vi "TRIG_CHAN_AUX_HAND.vi"(0 "VISA IN":refnum<visa-resource-name>, 1 "Aux":i32, 2 "Handshake":bool, 5 "error in":errorcluster, 7 "Channel":i32) -> (14 "VISA Out":refnum<visa-resource-name>, 19 "error out":errorcluster)   [LabVIEW 2018, in "PNA-X.lvlib"]
doc: "TRIGger:CHANnel<ch>:AUX<n>:HANDshake <bool> \n(Read-Write) Turns handshake ON / OFF. \nTo enable handshake, the main trigger enable must also be set using TRIG:CHAN:AUX:ENAB. \nWhen ON, PNA waits indefinitely for the input line to be asserted before continuing with the \nacquisition. When OFF, the PNA acquires data without waiting. \nParameters \n<ch> Any existing channel number. If unspecified, value is set to 1. \n<n> Rear panel connector used to send or receive signals. \nPNA-X - choose from 1 (AUX TRIG 1) or 2 (AUX TRIG 2) \nAll other models: choose 1. (BNC Trig I/O \nIf unspecified, value is set to 1. \n<bool> ON (or 1) - turns handshaking ON. \nOFF (or 0) - turns handshaking OFF. \nExamples TRIG:CHAN:AUX:HAND 1 \ntrigger:channel2:aux2:handshake off \nQuery Syntax TRIGger:CHANnel<ch>:AUX<n>:HANDshake? \nReturn Type Boolean \nDefault OFF"
uses:
  PNA-X.lvlib
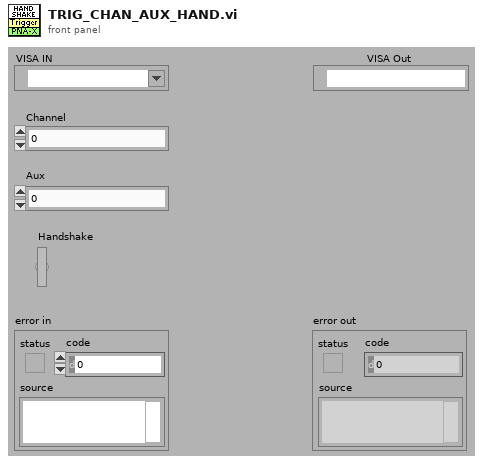
[diagram p1: front panel]
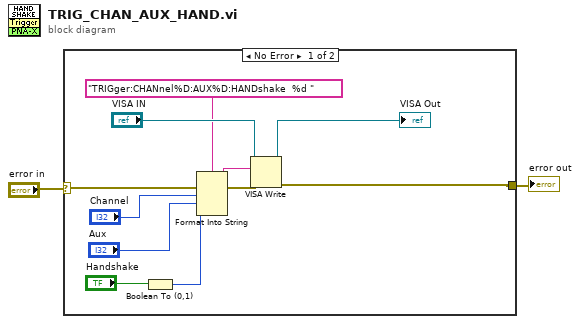
[diagram p0: block diagram]
diagram:
  n1 = case shown="No Error" "error in" {
    selector: "error in" -> [w13 w14]
    tunnel: [w8 w14] -> w1
    frame No Error {
      n2 = Boolean To (0,1)(Boolean="Handshake") -> (0, 1=w4:i16)
      n3 = Format Into String(format string="TRIGger:CHANnel%D:AUX%D:HANDshake  %d " ("Cmdline"), error in=w13, "Channel", "Aux", w4) -> (resulting string=w11:string, error out=w12:errorcluster)  [unwired: 1 in]
      n4 = VISA Write(VISA resource name="VISA IN", write buffer=w11, error in (no error)=w12) -> (VISA resource name out=→"VISA Out":refnum<visa-resource-name>, error out=w8:errorcluster)  [unwired: 1 out]
    }
    frame Error {
    }
  }
  "error out" <- w1
